vi "CLD 8 CSV file commands utility Exercise.vi"(8 "Error In":errorcluster) -> (0 "Error Out":errorcluster, 3 "Commands Out Array":T1[](array[typedef]))   [LabVIEW 2020]
doc: "CLD 8 exercise"
uses:
  CLD 8 Data Cluster.ctl
  <vilib>/Utility/file.llb/Read Delimited Spreadsheet (string).vi
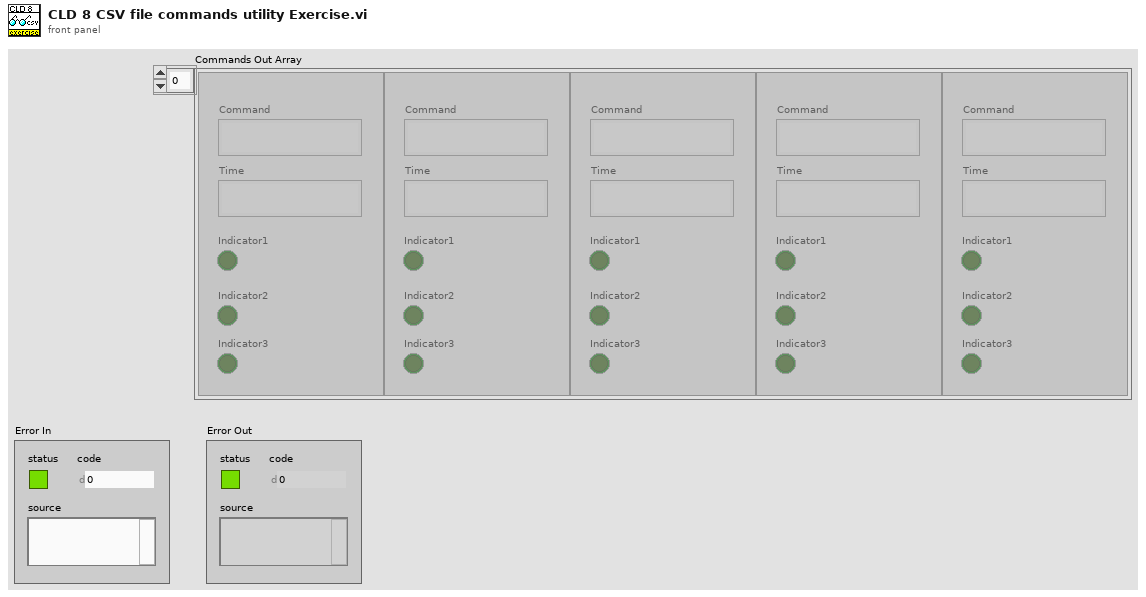
[diagram p1: front panel]
types:
  T1 = typedef "CLD 8 Data Cluster.ctl" = cluster{"Command":string, "Time":string, "Indicator1":bool, "Indicator2":bool, "Indicator3":bool}
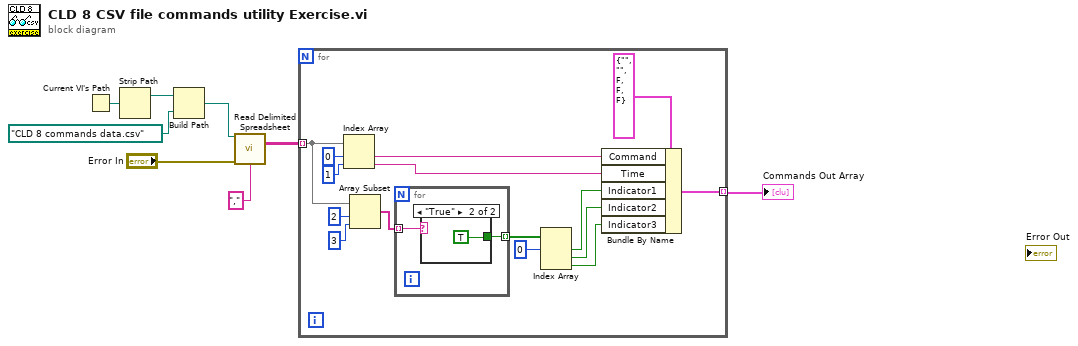
[diagram p0: block diagram]
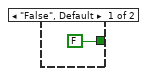
[diagram p2: hidden frame]
diagram:
  n1 = Current VI's Path() -> (path=w7:path)
  n2 = Strip Path(path=w7) -> (stripped path=w6:path)  [unwired: 1 out]
  n3 = Build Path(base path=w6, name or relative path=path "CLD 8 commands data.csv") -> (appended path=w4:path)
  n4 = call-poly <vilib>:"Read Delimited Spreadsheet.vi"("file path (dialog if empty)"=w4, "error in (no error)"="Error In", "delimiter (\\t)"="," ("delimiter (\\t)")) -> ("all rows"=w8:string[][])  [unwired: 7 in, 5 out]
  n5 = for {
    tunnel: [w22] -> w1 mode=indexing
    tunnel: w8 -> [w17] mode=indexing
    n6 = Index Array(array=w17, index #1=0 ("index"), index #2=1 ("index")) -> (element #1=w20:string, element #2=w19:string)
    n7 = Array Subset(array=w17, index=2, length=3) -> (w14:string[])
    n8 = for {
      tunnel: w14 -> [w25] mode=indexing
      tunnel: [w24] -> w13 mode=indexing
      n9 = case shown="\"True\"" w25 {
        tunnel: [FALSE TRUE] -> w24
        frame "False", Default {
        }
        frame "True" {
        }
      }
    }
    n10 = Index Array(array=w13, index #1=0 ("index")) -> (element #1=w11:bool, element #2=w10:bool, element #3=w9:bool)  [unwired: 2 in]
    n11 = Bundle By Name(cluster=T1 {"Command"="", "Time"="", "Indicator1"=FALSE, "Indicator2"=FALSE, "Indicator3"=FALSE} ("Cluster 3"), "Command"=w20, "Time"=w19, "Indicator1"=w11, "Indicator2"=w10, "Indicator3"=w9) -> (w22:T1)
  }
  "Commands Out Array" <- w1
